vi "FPGA_target_split_bit_information.vi"(1 "data in":u16 format="%01b") -> (0 "connector_data":T1)   [LabVIEW 2014]
doc: "splits a 32 bit number into a cluster of four bytes"
uses:
  FPGA_32BitPattern_data_type.ctl
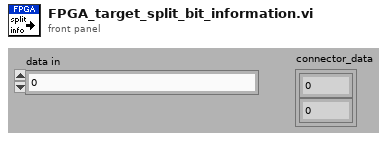
[diagram p1: front panel]
types:
  T1 = typedef "FPGA_32BitPattern_data_type.ctl" = cluster{"port0":u8, "port1":u8}
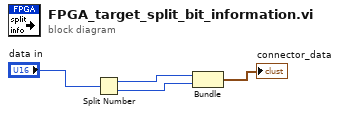
[diagram p0: block diagram]
diagram:
  n1 = Split Number(x="data in") -> (hi(x)=w4:u8, lo(x)=w3:u8)
  n2 = Bundle(w4, w3) -> (→"connector_data":cluster{u8, u8})  [unwired: 1 in]
